vi "util_stop_write.vi"(8 "error in (no error)":errorcluster, 11 "stop":bool) -> (0 "error out":errorcluster)   [LabVIEW 2015, in "lv-recipe-machine.lvlib" / "example_01.lvlib"]
uses:
  example_01.lvlib
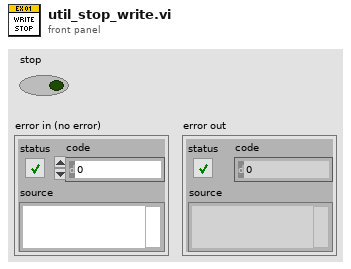
[diagram p1: front panel]
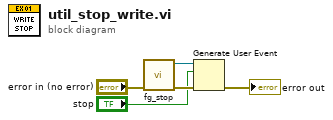
[diagram p0: block diagram]
diagram:
  n1 = call "fg_stop.vi"("error in (no error)"="error in (no error)") -> ("error out"=w4:errorcluster, "stop_event"=w5:refnum<user-event>)  [unwired: 9 in]
  n2 = Generate User Event(user event=w5, event data cluster="stop", error in=w4) -> (error out=→"error out":errorcluster)  [unwired: 1 in, 1 out]
